vi "Open and Configure Device.vi"(0 "USRP RIO Device":T17, 5 "reference frequency source":string(combo)="Internal", 7 "which bitfile":string(combo)="SyncPps", 9 "Wait for GPS Lock?":bool, 11 "error in":errorcluster, 12 "rx config":T5={"rf enable 0"=FALSE, "rf config 0"={"antenna"="RX2", "frequency"=2000000000.0, "lo frequency"=-1.0, "level"=0.0}, "rf enable 1"=FALSE, "rf config 1"={"antenna"="RX2", "frequency"=2000000000.0, "lo frequency"=-1.0, "level"=0.0}, "number of samples is finite"=TRUE, "sample rate"=10000000.0, "number of samples"=8192, "start trigger"=enum."Immediate"} {"sample rate" format="%#.3pS/s"; "rf config 1"."level" format="%#_gdBm"; "rf config 1"."lo frequency" format="%#.3pHz"; "rf config 1"."frequency" format="%#.3pHz"; "rf config 0"."level" format="%#_gdBm"; "rf config 0"."lo frequency" format="%#.3pHz"; "rf config 0"."frequency" format="%#.3pHz"}, 13 "tx config":T6={"rf enable 0"=FALSE, "rf config 0"={"antenna"="TX1", "frequency"=2000000000.0, "lo frequency"=-1.0, "level"=0.0}, "rf enable 1"=FALSE, "rf config 1"={"antenna"="TX1", "frequency"=2000000000.0, "lo frequency"=-1.0, "level"=0.0}, "number of samples is finite"=TRUE, "sample rate"=10000000.0, "number of samples"=8192, "start trigger"=enum."Immediate", "tone frequency"=100000.0} {"tone frequency" format="%#.3pHz"; "sample rate" format="%#.3pS/s"; "rf config 0"."level" format="%#_gdBm"; "rf config 0"."lo frequency" format="%#.3pHz"; "rf config 0"."frequency" format="%#.3pHz"; "rf config 1"."level" format="%#_gdBm"; "rf config 1"."lo frequency" format="%#.3pHz"; "rf config 1"."frequency" format="%#.3pHz"}, 14 "x":cdb[](array[numeric])) -> (2 "rx channels":T4={"rx config"={"rf enable 0"=FALSE, "rf config 0"={"antenna"="RX2", "frequency"=2000000000.0, "lo frequency"=-1.0, "level"=0.0}, "rf enable 1"=FALSE, "rf config 1"={"antenna"="RX2", "frequency"=2000000000.0, "lo frequency"=-1.0, "level"=0.0}, "number of samples is finite"=TRUE, "sample rate"=10000000.0, "number of samples"=8192, "start trigger"=enum."Immediate"}, "reference frequency source"="Internal", "rx.enabled channels"=[], "vertical range"=[], "rx.coerced configurations"={"coerced frequencies"=[], "coerced lo frequencies"=[], "coerced levels"=[], "coerced sample rates"=[]}} {"rx.coerced configurations"."coerced sample rates" format="%#.3pS/s"; "rx.coerced configurations"."coerced levels" format="%#.3gdBm"; "rx.coerced configurations"."coerced lo frequencies" format="%#.3pHz"; "rx.coerced configurations"."coerced frequencies" format="%#.3pHz"; "rx config"."sample rate" format="%#.3pS/s"; "rx config"."rf config 1"."level" format="%#_gdBm"; "rx config"."rf config 1"."lo frequency" format="%#.3pHz"; "rx config"."rf config 1"."frequency" format="%#.3pHz"; "rx config"."rf config 0"."level" format="%#_gdBm"; "rx config"."rf config 0"."lo frequency" format="%#.3pHz"; "rx config"."rf config 0"."frequency" format="%#.3pHz"; "vertical range" format="%#.3pVpp"}, 3 "tx channels":T3={"tx config"={"rf enable 0"=FALSE, "rf config 0"={"antenna"="TX1", "frequency"=2000000000.0, "lo frequency"=-1.0, "level"=0.0}, "rf enable 1"=FALSE, "rf config 1"={"antenna"="TX1", "frequency"=2000000000.0, "lo frequency"=-1.0, "level"=0.0}, "number of samples is finite"=TRUE, "sample rate"=10000000.0, "number of samples"=8192, "start trigger"=enum."Immediate", "tone frequency"=100000.0}, "reference frequency source"="Internal", "tx.enabled channels"=[], "I"=[], "Q"=[], "tx.coerced configurations"={"coerced frequencies"=[], "coerced lo frequencies"=[], "coerced levels"=[], "coerced sample rates"=[]}} {"tx.coerced configurations"."coerced sample rates" format="%#.3pS/s"; "tx.coerced configurations"."coerced levels" format="%#.3gdBm"; "tx.coerced configurations"."coerced lo frequencies" format="%#.3pHz"; "tx.coerced configurations"."coerced frequencies" format="%#.3pHz"; "tx config"."tone frequency" format="%#.3pHz"; "tx config"."sample rate" format="%#.3pS/s"; "tx config"."rf config 0"."level" format="%#_gdBm"; "tx config"."rf config 0"."lo frequency" format="%#.3pHz"; "tx config"."rf config 0"."frequency" format="%#.3pHz"; "tx config"."rf config 1"."level" format="%#_gdBm"; "tx config"."rf config 1"."lo frequency" format="%#.3pHz"; "tx config"."rf config 1"."frequency" format="%#.3pHz"}, 4 "niUsrpRio Session (out)":T8 {"FPGA Data Clock Rate" format="%#.3pHz"; "Data Clock Rate" format="%#.3pHz"; "Characterization Data"."Frequencies [Hz]" format="%#_6p"; "EEPROM Characterization Header"."Pointer to Device Data Header" format="%x"; "EEPROM Characterization Header"."Checksum" format="%x"; "Device Data Header"."Pointer to Characterization Data" format="%x"; "Device Data Header"."Checksum" format="%x"; "EEPROM Header"."Pointer to User Header" format="%x"; "EEPROM Header"."Pointer to Factory Header" format="%x"; "EEPROM Header"."Product Code" format="%x"; "EEPROM Header"."Checksum" format="%x"}, 6 "rx.coerced configurations":T7 {"coerced sample rates" format="%#.3pS/s"; "coerced levels" format="%#.3gdBm"; "coerced lo frequencies" format="%#.3pHz"; "coerced frequencies" format="%#.3pHz"}, 8 "tx.coerced configurations":T7 {"coerced sample rates" format="%#.3pS/s"; "coerced levels" format="%#.3gdBm"; "coerced lo frequencies" format="%#.3pHz"; "coerced frequencies" format="%#.3pHz"}, 15 "error out":errorcluster)   [LabVIEW 2015]
uses:
  <vilib>/userdefined/Silver/nirio_resource_slv.ctl
  <instrlib>/niUsrpRio/Config/v1/Host/Public/niUsrpRio Session.ctl
  <instrlib>/_niInstr/Register Bus/v0/Host/Public/Register Bus Session.ctl
  <instrlib>/_niInstr/Register Bus/v0/Host/Private/Session Data.ctl
  <instrlib>/niUsrpRio/Config/v1/Host/Private/DB Queue Reference.ctl
  <instrlib>/niUsrpRio/Config/v1/Host/Private/Daughterboard Data.ctl
  <instrlib>/niUsrpRio/Config/v1/Host/Private/ATR state data.ctl
  <instrlib>/niUsrpRio/Config/v1/Host/Public/EEPROM Header.ctl
  <instrlib>/niUsrpRio/Config/v1/Host/Public/EEPROM Device Data Header.ctl
  <instrlib>/niUsrpRio/Config/v1/Host/Public/EEPROM Characterization Header.ctl
  <instrlib>/niUsrpRio/Config/v1/Host/Public/Characterization Data.ctl
  <instrlib>/niUsrpRio/Config/v1/Host/Public/IQ Imbalance.ctl
  Start Trigger.ctl
  <instrlib>/niUsrpRio/Config/v1/Host/Public/What to Query for.ctl
  Supporting Files/Global Vars.vi
  <instrlib>/niUsrpRio/Config/v1/Host/niUsrpRio Config v1 Host.lvlib
  <instrlib>/_niInstr/Register Bus/v0/Host/niInstr Register Bus v0 Host.lvlib
panel:
  in  "?":T1=enum."GPS Lock Status"
  in  "scope":string
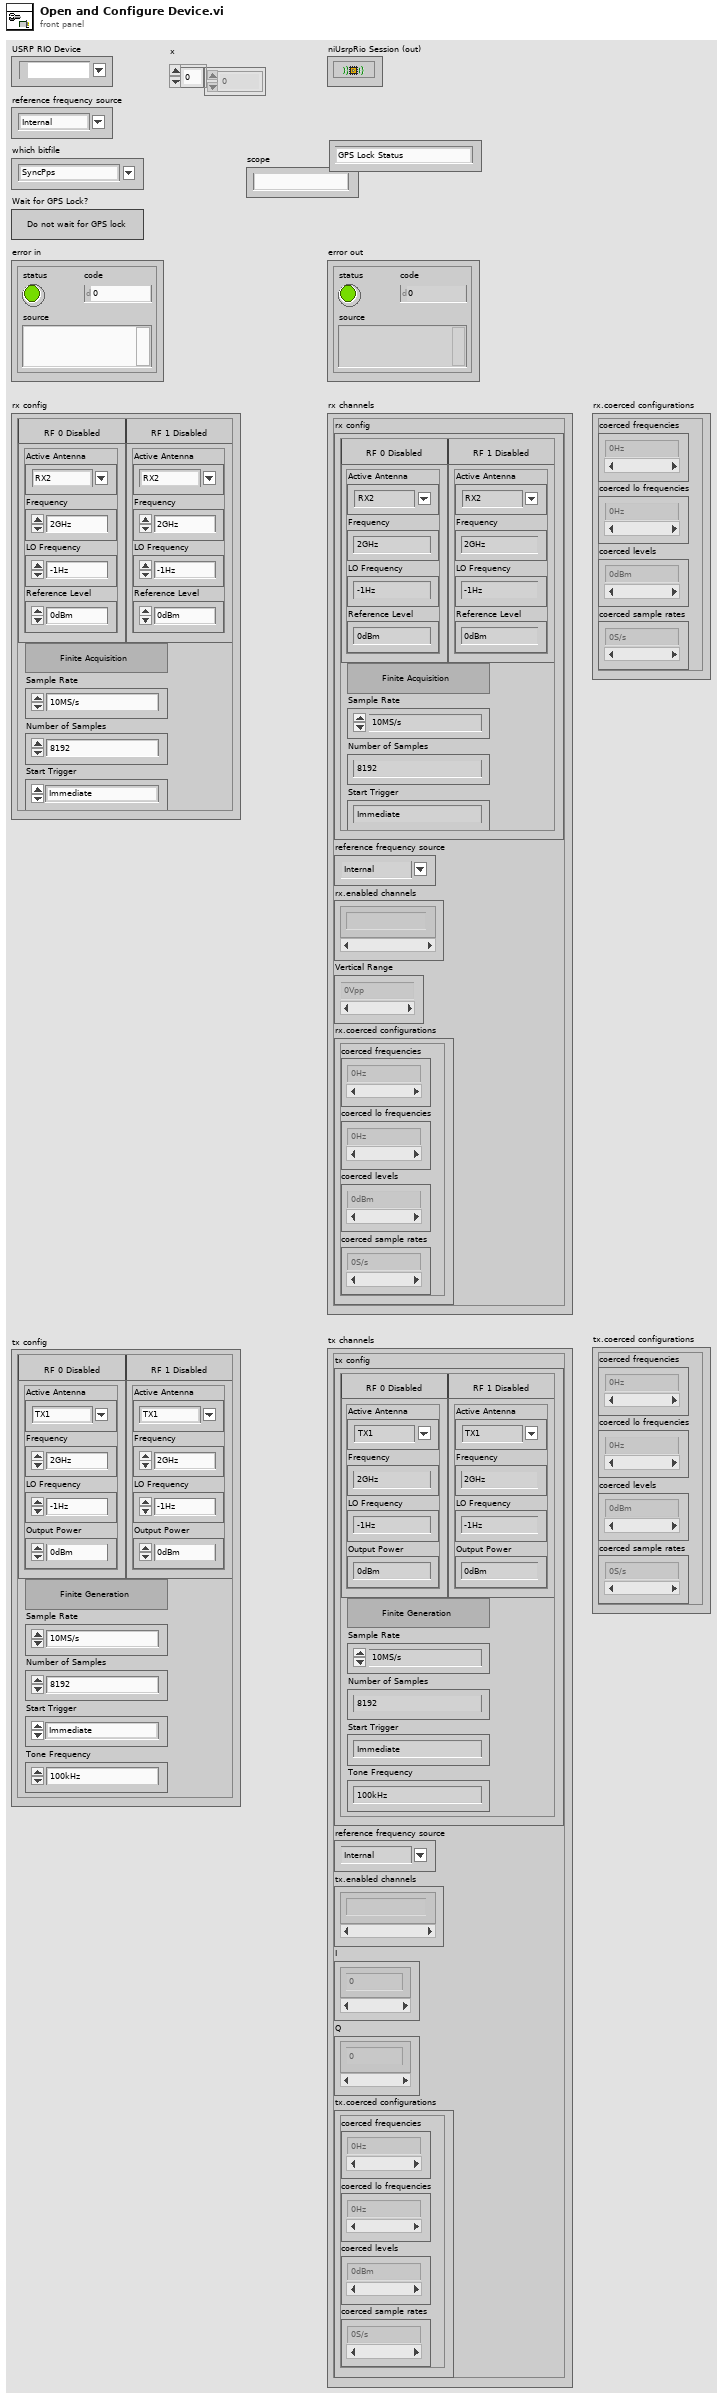
[diagram p1: front panel]
types:
  T1 = typedef "niUsrpRio Config v1 Host.lvlib/What to Query for.ctl" = enum16{"Clock Chip Lock Status", "Clock Chip Ever Unlocked", "LO Lock Status", "GPS Lock Status", "GPS Ever Unlocked", "DRAM Ready Status", "DAC PLL Lock Status", "DAC Sync Lock Status", "Data Clock PLL Lock Status", "Data Clock PLL Ever Unlocked", "ADC Clock PLL Lock Status", "ADC Clock PLL Ever Unlocked", "ADC Data Valid Status", "ADC Data Ever Invalid"}
  T2 = typedef "Start Trigger.ctl" = enum8{"Software", "Digital Edge", "Rx Start Trigger", "Tx Start Trigger", "Immediate", "Future Time Event"}
  T3 = cluster{"tx config":cluster{"rf enable 0":bool, "rf config 0":cluster{"antenna":string, "frequency":dbl, "lo frequency":dbl, "level":dbl}, "rf enable 1":bool, "rf config 1":cluster{"antenna":string, "frequency":dbl, "lo frequency":dbl, "level":dbl}, "number of samples is finite":bool, "sample rate":dbl, "number of samples":u32, "start trigger":T2, "tone frequency":dbl}, "reference frequency source":string, "tx.enabled channels":string[], "I":i16[], "Q":i16[], "tx.coerced configurations":cluster{"coerced frequencies":dbl[], "coerced lo frequencies":dbl[], "coerced levels":dbl[], "coerced sample rates":dbl[]}}
  T4 = cluster{"rx config":cluster{"rf enable 0":bool, "rf config 0":cluster{"antenna":string, "frequency":dbl, "lo frequency":dbl, "level":dbl}, "rf enable 1":bool, "rf config 1":cluster{"antenna":string, "frequency":dbl, "lo frequency":dbl, "level":dbl}, "number of samples is finite":bool, "sample rate":dbl, "number of samples":u32, "start trigger":T2}, "reference frequency source":string, "rx.enabled channels":string[], "vertical range":dbl[], "rx.coerced configurations":cluster{"coerced frequencies":dbl[], "coerced lo frequencies":dbl[], "coerced levels":dbl[], "coerced sample rates":dbl[]}}
  T5 = cluster{"rf enable 0":bool, "rf config 0":cluster{"antenna":string, "frequency":dbl, "lo frequency":dbl, "level":dbl}, "rf enable 1":bool, "rf config 1":cluster{"antenna":string, "frequency":dbl, "lo frequency":dbl, "level":dbl}, "number of samples is finite":bool, "sample rate":dbl, "number of samples":u32, "start trigger":T2}
  T6 = cluster{"rf enable 0":bool, "rf config 0":cluster{"antenna":string, "frequency":dbl, "lo frequency":dbl, "level":dbl}, "rf enable 1":bool, "rf config 1":cluster{"antenna":string, "frequency":dbl, "lo frequency":dbl, "level":dbl}, "number of samples is finite":bool, "sample rate":dbl, "number of samples":u32, "start trigger":T2, "tone frequency":dbl}
  T7 = cluster{"coerced frequencies":dbl[], "coerced lo frequencies":dbl[], "coerced levels":dbl[], "coerced sample rates":dbl[]}
  T8 = typedef "niUsrpRio Config v1 Host.lvlib/niUsrpRio Session.ctl" = cluster{"FPGA Interface":refnum<k20>, "RIO Interface Number":u32, "Data Clock Rate":u32, "FPGA Data Clock Rate":u32, "Global Settings Register Bus":T9, "Radio 0 Settings Register Bus":T9, "Radio 1 Settings Register Bus":T9, "Radio Settings Bus Semaphore":T10, "DB Queues":T11[], "Characterization Data Valid?":bool, "EEPROM Header":T12, "Device Data Header":T13, "EEPROM Characterization Header":T14, "Characterization Data":T15[], "FPGA Current Version":u32, "FPGA Oldest Compatible Version":u32, "Fixed Logic Current Version":u32, "Fixed Logic Oldest Compatible Version":u32, "FPGA Radio Settings Bus Current Version":u32, "FPGA Radio Settings Bus Oldest Compatible Version":u32, "FPGA Board Config Current Version":u32, "FPGA Board Config Oldest Compatible Version":u32}
  T9 = typedef "niInstr Register Bus v0 Host.lvlib/Register Bus Session.ctl" = refnum<queue>
  T10 = typedef "Semaphore RefNum" = refnum<k1>
  T11 = typedef "niUsrpRio Config v1 Host.lvlib/DB Queue Reference.ctl" = refnum<queue>
  T12 = typedef "niUsrpRio Config v1 Host.lvlib/EEPROM Header.ctl" = cluster{"Checksum":u32, "Product Code":u16, "Hardware Current Version":u16, "Hardware Oldest Compatible Version":u16, "EEPROM Map Current Version":u16, "EEPROM Map Oldest Compatible Version":u16, "User Password":string, "Pointer to Factory Header":u32, "Pointer to User Header":u32, "Recommended Interval":u16, "Number of Reserved Bytes":i32, "Number of Daughterboards":u8, "Daughterboard IDs":u16[], "Daughterboard Serial Numbers":string[]}
  T13 = typedef "niUsrpRio Config v1 Host.lvlib/EEPROM Device Data Header.ctl" = cluster{"Checksum":u32, "Number of Channels":u8, "Number of Gain Settings":u16[], "Pointer to Characterization Data":u32[], "Number of Reserved Bytes":i32, "Number of Frequencies":u16[]}
  T14 = typedef "niUsrpRio Config v1 Host.lvlib/EEPROM Characterization Header.ctl" = cluster{"Checksum":u32, "Date":timestamp, "Temperature":sgl, "Misc. Info":string, "Pointer to Device Data Header":u32, "Number of Reserved Bytes":i32}
  T15 = typedef "niUsrpRio Config v1 Host.lvlib/Characterization Data.ctl" = cluster{"Gains[dB]":dbl[], "Frequencies [Hz]":dbl[], "IQ Imbalance Table":T16[], "Measured Gains[dB]":dbl[][]}
  T16 = typedef "niUsrpRio Config v1 Host.lvlib/IQ Imbalance.ctl" = cluster{"Gain Imbalance [linear]":dbl, "Phase Imbalance [radians]":dbl, "Offset":cdb}
  T17 = typedef "nirio_resource_slv.ctl" = tag
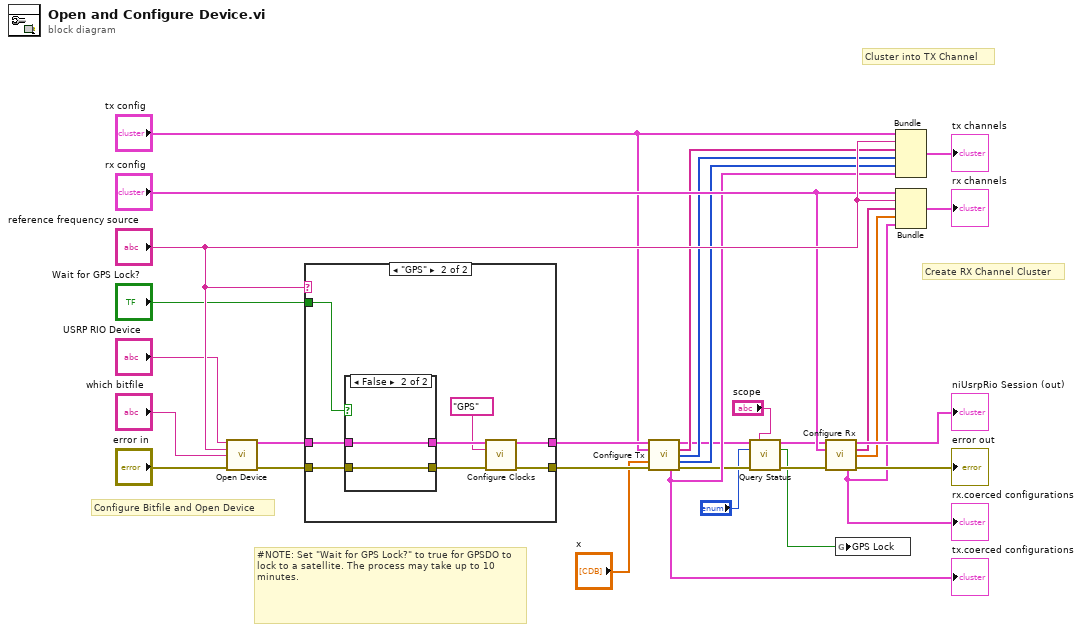
[diagram p0: block diagram]
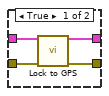
[diagram p3: hidden frame]
diagram:
  # "Configure Bitfile and Open Device"
  # "Create RX Channel Cluster"
  # "Cluster into TX Channel"
  # "#NOTE: Set \"Wait for GPS Lock?\" to true for GPSDO to lock to a satellite. The process may take up to 10 minutes."
  n1 = call "Open Device.vi"("USRP RIO device"="USRP RIO Device", "Reference Frequency Source"="reference frequency source", "which bitfile"="which bitfile", "error in"="error in") -> ("niUsrpRio Session (out)"=w21:T8, "error out"=w22:errorcluster)  [unwired: 10 in]
  n2 = case shown="\"GPS\"" "reference frequency source" {
    tunnel: w21 -> [w32 w40]
    tunnel: [w32 w35] -> w28
    tunnel: [w31 w37] -> w20
    tunnel: w22 -> [w31 w39]
    tunnel: "Wait for GPS Lock?" -> [_ w33]
    frame Default {
    }
    frame "GPS" {
      n3 = case shown="False" w33 {
        tunnel: w40 -> [w42 w46]
        tunnel: [w44 w46] -> w36
        tunnel: [w43 w45] -> w38
        tunnel: w39 -> [w41 w45]
        frame True {
          n4 = call "Lock to GPS.vi"("niUsrpRio Session"=w42, "error in"=w41) -> ("niUsrpRio Session (out)"=w44:T8, "error out"=w43:errorcluster)  [unwired: 12 in]
        }
        frame False {
        }
      }
      n5 = call "Configure Clocks.vi"("niUsrpRio Session"=w36, "Reference Frequency Source"="GPS", "error in"=w38) -> ("niUsrpRio Session (out)"=w35:T8, "error out"=w37:errorcluster)  [unwired: 11 in]
    }
  }
  n6 = call "Configure Tx.vi"("niUsrpRio Session"=w28, "tx config"="tx config", "x"="x", "error in"=w20) -> ("niUsrpRio Session (out)"=w8:T8, "tx.enabled channels"=w16:string[], "I"=w15:i16[], "Q"=w14:i16[], "tx.coerced configurations"=w11:T7, "error out"=w7:errorcluster)  [unwired: 6 in]
  "tx.coerced configurations" <- w11
  n7 = call <instrlib>:"Query Status.vi"("niUsrpRio Session"=w8, "scope"="scope", "What to Query for"="?", "error in"=w7) -> ("niUsrpRio Session (out)"=w5:T8, "Status"=w4:bool, "error out"=w6:errorcluster)  [unwired: 9 in]
  n8 = call "Configure Rx.vi"("niUsrpRio Session"=w5, "rx config"="rx config", "error in"=w6) -> ("niUsrpRio Session (out)"=→"niUsrpRio Session (out)":T8, "rx.enabled channels"=w18:string[], "vertical range"=w17:dbl[], "rx.coerced configurations"=w10:T7, "error out"=→"error out":errorcluster)  [unwired: 8 in]
  "rx.coerced configurations" <- w10
  n9 = global write "Global Vars.vi" "GPS Lock"(w4) -> ()
  n10 = Bundle("tx config"="tx config", "reference frequency source"="reference frequency source", "tx.enabled channels"=w16, "I"=w15, "Q"=w14, "tx.coerced configurations"=w11) -> (→"tx channels":T3)  [unwired: 1 in]
  n11 = Bundle("rx config"="rx config", "reference frequency source"="reference frequency source", "rx.enabled channels"=w18, "vertical range"=w17, "rx.coerced configurations"=w10) -> (→"rx channels":T4)  [unwired: 1 in]
